vi "Update Panel (Type).vi"(8 "error in (no error)":errorcluster, 9 "Ctl Refnum":refnum<vi>, 10 "Control Type":string, 11 "Editor in":refnum<class "Editor.lvclass">) -> (0 "error out":errorcluster, 3 "Editor out":refnum<class "Editor.lvclass">)   [LabVIEW 2020, in "VolatusGUIEditor.lvlib" / "Editor.lvclass"]
uses:
  Editor.lvclass
  lv-oopanel/OOPanel/Manager/Manager.lvclass
  VolatusGUIEditorCore/ElementEditorPanel/ElementEditorPanel.lvclass
  C:/dev/lv20CE/relink/lv-oopanel/OOPanel/Panel/Panel.lvclass
  C:/dev/lv20CE/relink/volatus-gui-controls/VolatusGUIControls/ElementEditorPanel/ElementEditorPanel.lvclass
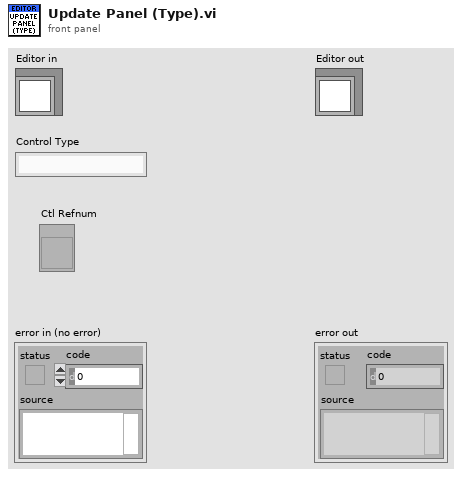
[diagram p1: front panel]
types:
  T1 = map{string, refnum<class "ElementEditorPanel.lvclass">}
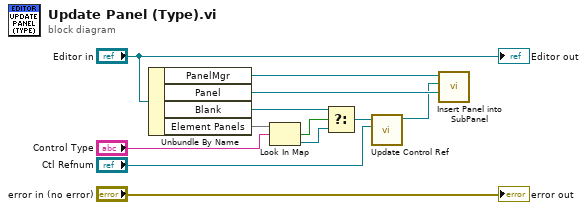
[diagram p0: block diagram]
diagram:
  n1 = Unbundle By Name("Editor in") -> ("PanelMgr"=w11:refnum<class "Manager.lvclass">, "Panel"=w10:refnum<vi>, "Blank"=w9:refnum<class "ElementEditorPanel.lvclass">, "Element Panels"=w6:T1)
  n2 = Look In Map(map=w6, key="Control Type") -> (key not found?=w4:bool, value=w3:refnum<class "ElementEditorPanel.lvclass">)  [unwired: 1 in]
  n3 = Select(t=w9, s=w4, f=w3) -> (s? t:f=w8:refnum<class "ElementEditorPanel.lvclass">)
  n4 = call "Update Control Ref.vi"("Ctl Refnum"="Ctl Refnum", "ElementEditorPanel in"=w8) -> ("ElementEditorPanel out"=w2:refnum<class "ElementEditorPanel.lvclass">)  [unwired: 8 in, 1 out]
  n5 = call "Insert Panel into SubPanel.vi"("SubPanel"=w10, "Panel In"=w2, "Manager in"=w11) -> ()  [unwired: 6 in, 3 out]
  "error out" <- "error in (no error)"
  "Editor out" <- "Editor in"
